vi "Init.vi"(8 "error in (no error)":errorcluster, 9 "Config File Path":path=path "", 10 "Name":string, 11 "Slave Test Runner In":refnum<class "Slave Test Runner.lvclass">) -> (0 "error out":errorcluster, 3 "Slave Test Runner Out":refnum<class "Slave Test Runner.lvclass">)   [LabVIEW 2020, in "Slave Test Runner.lvclass"]
uses:
  Slave Test Runner.lvclass
  Test Case/LUnit Test Case.lvclass
  Slave Test Runner.lvclass/Slave Test Runner.ctl
  Application Framework/Process Classes/Process/Process.lvclass
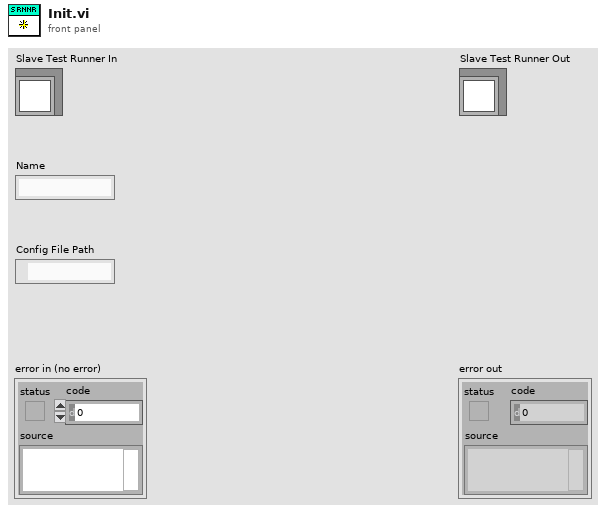
[diagram p1: front panel]
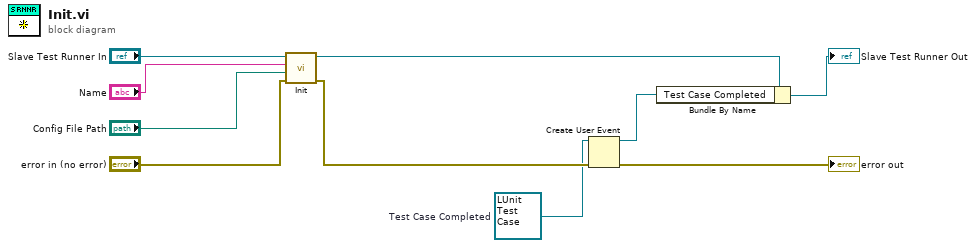
[diagram p0: block diagram]
diagram:
  w2 = refnum<class "LUnit Test Case.lvclass"> refnum  # Test Case Completed
  n1 = call-parent "Init.vi"("error in (no error)"="error in (no error)", "Config File Path"="Config File Path", "Name"="Name", "Process In"="Slave Test Runner In") -> ("error out"=w6:errorcluster, "Process Out"=w9:refnum<class "Slave Test Runner.lvclass">)  [unwired: 6 in]
  n2 = Create User Event(user event datatype=w2, error in=w6) -> (user event=w1:refnum<user-event>, error out=→"error out":errorcluster)
  n3 = Bundle By Name(cluster=w9, "Test Case Completed"=w1) -> (→"Slave Test Runner Out":refnum<class "Slave Test Runner.lvclass">)
